vi "NOMEDECENTE (SubVI).vi"(0 "In source":refnum<visa-resource-name>, 1 "error in RLC":errorcluster, 5 "RLC in":refnum<visa-resource-name>, 7 "Current":dbl, 9 "Field":dbl, 11 "error in source":errorcluster, 12 "milliseconds to wait":u32=1000) -> (2 "VISA resource name out 2":refnum<visa-resource-name>, 3 "Modulo 2":dbl format="%^.4e", 4 "VISA Refnum out":refnum<visa-resource-name>, 6 "error out 3":errorcluster, 8 "Fase 2":dbl format="%^.4e", 10 "Fase":cluster{"X":dbl[], "Y":dbl[]}[](graph) caption="XY Graph", 13 "Modulo":cluster{"X":dbl[], "Y":dbl[]}[](graph) caption="XY Graph", 14 "Data Status":bool=TRUE, 15 "error out":errorcluster)   [LabVIEW 2015]
uses:
  <vilib>/Analysis/baseanly.llb/Mean (DBL).vi
  <instrlib>/Agilent E364X Series/Agilent E364X Series.lvlib
  <instrlib>/Agilent 428X Series/Agilent 428X Series.lvlib
  <vilib>/Analysis/NI_AALBase.lvlib
panel:
  out "fase":dbl
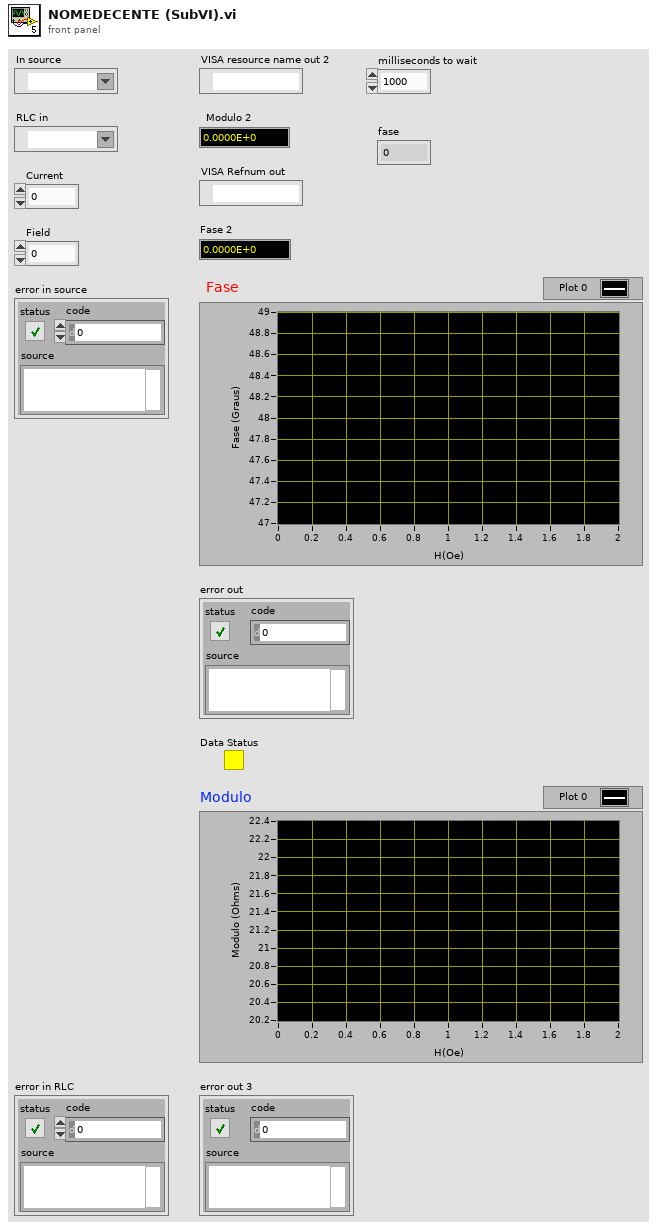
[diagram p1: front panel]
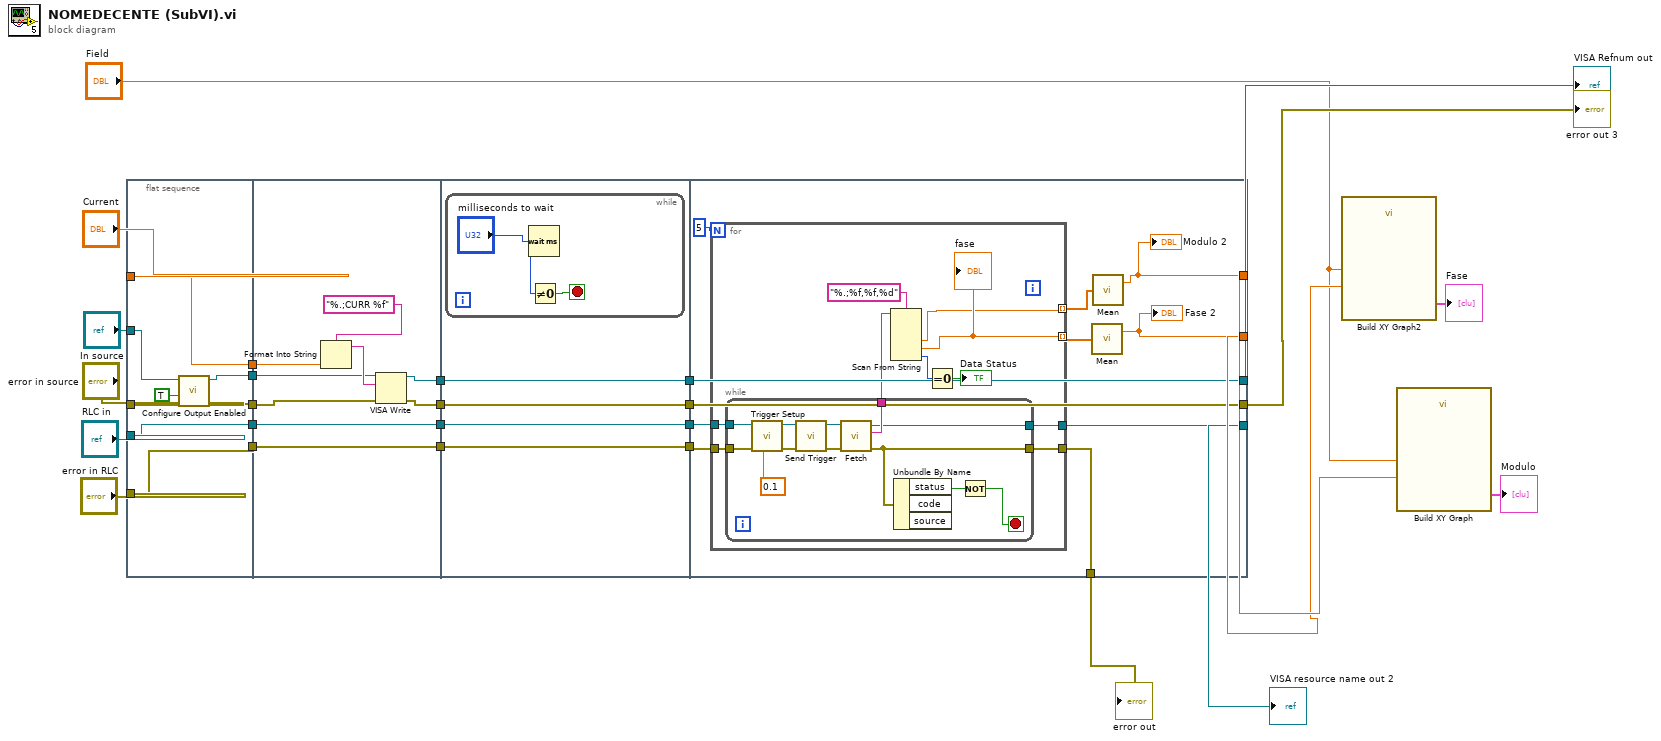
[diagram p0: block diagram]
diagram:
  n1 = flat-sequence {
    tunnel: "Current" -> [w35]
    tunnel: "In source" -> [w34]
    tunnel: "error in source" -> [w33]
    tunnel: [w31] -> w27
    tunnel: [w32] -> w26
    tunnel: [w35] -> w25
    tunnel: "RLC in" -> [w29]
    tunnel: [w29] -> w24
    tunnel: [w28] -> w23
    tunnel: "error in RLC" -> [w28]
    tunnel: w27 -> [w42]
    tunnel: w26 -> [w41]
    tunnel: w25 -> [w38]
    tunnel: [w40] -> w22
    tunnel: [w39] -> w21
    tunnel: [w37] -> w20
    tunnel: w24 -> [w37]
    tunnel: [w36] -> w19
    tunnel: w23 -> [w36]
    tunnel: w22 -> [w48]
    tunnel: [w48] -> w18
    tunnel: w21 -> [w47]
    tunnel: [w47] -> w17
    tunnel: w20 -> [w46]
    tunnel: [w46] -> w16
    tunnel: w19 -> [w45]
    tunnel: [w45] -> w15
    tunnel: [w61] -> w10
    tunnel: [w62] -> w6
    tunnel: w18 -> [w62]
    tunnel: w17 -> [w61]
    tunnel: w16 -> [w59]
    tunnel: w15 -> [w58]
    tunnel: [w53] -> w8
    tunnel: [w52] -> w9
    tunnel: [w57] -> w2
    tunnel: [w56] -> w1
    frame #0 {
      n2 = call <instrlib>:"Configure Output Enabled.vi"("error in (no error)"=w33, "Output Enabled (F: Off)"=TRUE, "VISA resource name"=w34) -> ("error out"=w31:errorcluster, "VISA resource name out"=w32:refnum<visa-resource-name>)  [unwired: 7 in]
    }
    frame #1 {
      n3 = Format Into String(format string="%.;CURR %f", w38) -> (resulting string=w44:string)  [unwired: 2 in, 1 out]
      n4 = VISA Write(VISA resource name=w41, write buffer=w44, error in (no error)=w42) -> (VISA resource name out=w40:refnum<visa-resource-name>, error out=w39:errorcluster)  [unwired: 1 out]
    }
    frame #2 {
      n5 = while {
        stop <- w50 stop-if-true
        n6 = Wait (ms)(milliseconds to wait="milliseconds to wait") -> (millisecond timer value=w51:u32)
        n7 = Not Equal To 0?(x=w51) -> (x != 0?=w50:bool)
      }
    }
    frame #3 {
      n8 = for {
        N: 5 -> [_]
        tunnel: [w68] -> w54 mode=indexing
        tunnel: [w67] -> w55 mode=indexing
        tunnel: w59 -> [w66]
        tunnel: w58 -> [w65]
        tunnel: [w64] -> w57
        tunnel: [w63] -> w56
        n9 = while {
          tunnel: [w83] -> w72
          tunnel: w66 -> [w76]
          tunnel: w65 -> [w75]
          tunnel: [w74] -> w64
          tunnel: [w73] -> w63
          stop <- w77 stop-if-true
          n10 = call <instrlib>:"Trigger Setup.vi"("Delay Value (s) (0.0)"=0.1, "error in (no error)"=w75, "VISA resource name"=w76) -> ("error out"=w79:errorcluster, "VISA resource name out"=w80:refnum<visa-resource-name>)  [unwired: 7 in]
          n11 = call <instrlib>:"Send Trigger.vi"("error in (no error)"=w79, "VISA resource name"=w80) -> ("error out"=w82:errorcluster, "VISA resource name out"=w84:refnum<visa-resource-name>)  [unwired: 8 in]
          n12 = call <instrlib>:"Fetch.vi"("error in (no error)"=w82, "VISA resource name"=w84) -> ("error out"=w73:errorcluster, "Returned Data"=w83:string, "VISA resource name out"=w74:refnum<visa-resource-name>)  [unwired: 7 in]
          n13 = Unbundle By Name(w73) -> ("status"=w78:bool)  [unwired: 2 out]
          n14 = Not(x=w78) -> (.not. x?=w77:bool)
        }
        n15 = Scan From String(format string="%.;%f,%f,%d", input string=w72) -> (output 1=w67:dbl, output 2=w68:dbl, output 3=w69:i32)  [unwired: 5 in, 3 out]
        "fase" <- w68
        n16 = Equal To 0?(x=w69) -> (x = 0?=→"Data Status":bool)
      }
      n17 = call-poly <vilib>:"Mean.vi"("X"=w54) -> ("mean"=w53:dbl)  [unwired: 1 out]
      "Fase 2" <- w53
      n18 = call-poly <vilib>:"Mean.vi"("X"=w55) -> ("mean"=w52:dbl)  [unwired: 1 out]
      "Modulo 2" <- w52
    }
  }
  n19 = call "Build XY Graph2"("Y Input"=w8, "X Input"="Field") -> ("XY Graph"=→"Fase":cluster{"X":dbl[], "Y":dbl[]}[])  [unwired: 8 in, 1 out]
  n20 = call "Build XY Graph"("Y Input"=w9, "X Input"="Field") -> ("XY Graph"=→"Modulo":cluster{"X":dbl[], "Y":dbl[]}[])  [unwired: 8 in, 1 out]
  "error out 3" <- w10
  "error out" <- w1
  "VISA resource name out 2" <- w2
  "VISA Refnum out" <- w6
